vi "flow_control.vi"(10 "Output channel (for flowing)":tag, 11 "Pulse amp (V)":dbl) -> ()   [LabVIEW 2018]
uses:
  <vilib>/DAQmx/write.llb/DAQmx Write (Analog DBL 1Chan 1Samp).vi
  <vilib>/DAQmx/create/channels.llb/DAQmx Create Channel (AO-Voltage-Basic).vi
  <vilib>/DAQmx/miscellaneous.llb/DAQmx Fill In Error Info.vi
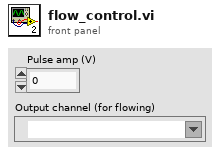
[diagram p1: front panel]
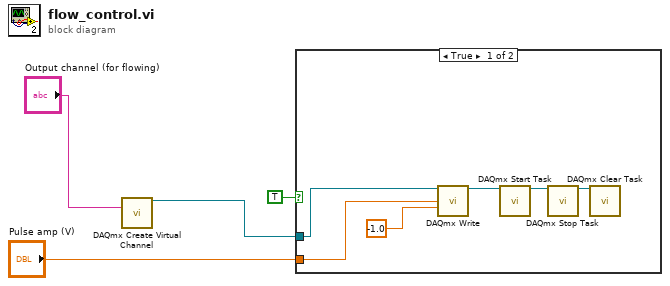
[diagram p0: block diagram]
diagram:
  n1 = call-poly <vilib>:"DAQmx Create Virtual Channel.vi"("physical channels"="Output channel (for flowing)") -> ("task out"=w3:refnum<k21>)  [unwired: 13 in, 1 out]
  n2 = case shown="True" TRUE {
    tunnel: "Pulse amp (V)" -> [w9 _]
    tunnel: w3 -> [w8 _]
    frame True {
      n3 = call-poly <vilib>:"DAQmx Write.vi"("task/channels in"=w8, "data"=w9, "timeout"=-1.0) -> ("task out"=w10:refnum<k21>)  [unwired: 10 in, 2 out]
      n4 = call <vilib>:"DAQmx Start Task.vi"("task/channels in"=w10) -> ("task out"=w6:refnum<k21>)  [unwired: 13 in, 1 out]
      n5 = call <vilib>:"DAQmx Stop Task.vi"("task/channels in"=w6) -> ("task out"=w7:refnum<k21>)  [unwired: 13 in, 1 out]
      n6 = call <vilib>:"DAQmx Clear Task.vi"("task in"=w7) -> ()  [unwired: 14 in, 1 out]
    }
    frame False {
    }
  }
